vi "Read Shared Variables Host.vi"(8 "error in (no error)":errorcluster, 11 "Shared Variable References":T1) -> (0 "error out":errorcluster, 2 "Current Values":T3, 3 "Shared Variable References Out":T1)   [LabVIEW 2014]
doc: "This VI reads the values in the application shared variables and passes those values out in a cluster."
uses:
  Custom Controls/Display State.ctl
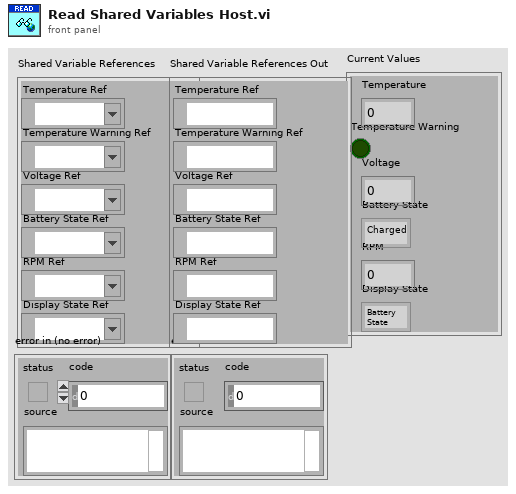
[diagram p1: front panel]
types:
  T1 = cluster{"Temperature Ref":refnum<k21>, "Temperature Warning Ref":refnum<k21>, "Voltage Ref":refnum<k21>, "Battery State Ref":refnum<k21>, "RPM Ref":refnum<k21>, "Display State Ref":refnum<k21>}
  T2 = typedef "Display State.ctl" = enum16{"Battery State", "RPM", "Temp", "Voltage"}
  T3 = cluster{"Temperature":fxp<+/-,32,13>, "Temperature Warning":bool, "Voltage":fxp<+/-,24,5>, "Battery State":enum16{"Charged", "Running", "Low Batt"}, "RPM":fxp<+,32,16>, "Display State":T2}
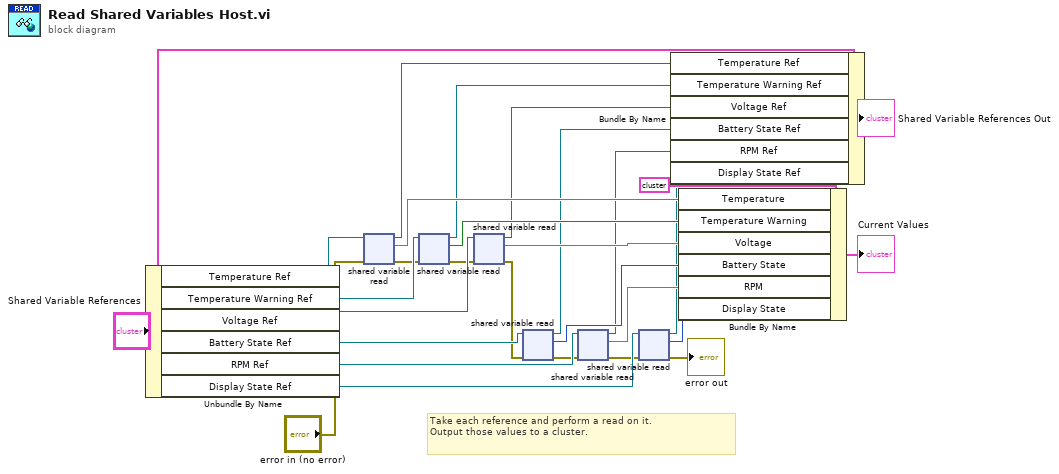
[diagram p0: block diagram]
diagram:
  # "Take each reference and perform a read on it.\nOutput those values to a cluster."
  n1 = Unbundle By Name("Shared Variable References") -> ("Temperature Ref"=w29:refnum<k21>, "Temperature Warning Ref"=w28:refnum<k21>, "Voltage Ref"=w27:refnum<k21>, "Battery State Ref"=w26:refnum<k21>, "RPM Ref"=w25:refnum<k21>, "Display State Ref"=w24:refnum<k21>)
  n2 = shared-variable-read(w29, "error in (no error)") -> (w7:refnum<k21>, w22:errorcluster, w16:fxp<+/-,32,13>)  [unwired: 1 out]
  n3 = shared-variable-read(w28, w22) -> (w6:refnum<k21>, w21:errorcluster, w15:bool)  [unwired: 1 out]
  n4 = shared-variable-read(w27, w21) -> (w5:refnum<k21>, w20:errorcluster, w14:fxp<+/-,24,5>)  [unwired: 1 out]
  n5 = shared-variable-read(w26, w20) -> (w4:refnum<k21>, w19:errorcluster, w13:enum16{"Charged", "Running", "Low Batt"})  [unwired: 1 out]
  n6 = shared-variable-read(w25, w19) -> (w3:refnum<k21>, w18:errorcluster, w12:fxp<+,32,16>)  [unwired: 1 out]
  n7 = shared-variable-read(w24, w18) -> (w2:refnum<k21>, →"error out":errorcluster, w11:T2)  [unwired: 1 out]
  n8 = Bundle By Name(cluster="Shared Variable References", "Temperature Ref"=w7, "Temperature Warning Ref"=w6, "Voltage Ref"=w5, "Battery State Ref"=w4, "RPM Ref"=w3, "Display State Ref"=w2) -> (→"Shared Variable References Out":T1)
  n9 = Bundle By Name(cluster=T3 {"Temperature"=0.0, "Temperature Warning"=FALSE, "Voltage"=0.0, "Battery State"=enum."Charged", "RPM"=0.0, "Display State"=enum."RPM"}, "Temperature"=w16, "Temperature Warning"=w15, "Voltage"=w14, "Battery State"=w13, "RPM"=w12, "Display State"=w11) -> (→"Current Values":T3)
